vi "Save.vi"(8 "error in":errorcluster, 10 "file path":path, 11 "cRIO repo in":refnum<class "database file.lvclass">) -> (0 "error out":errorcluster, 3 "cRIO repo out":refnum<class "database file.lvclass">)   [LabVIEW 2013, in "database file.lvclass"]
doc: "Calls the Read Tree VI to have an updated version of the Repo and then saves the repo information into the XML file."
uses:
  database file.lvclass
  database file.lvclass/database file.ctl
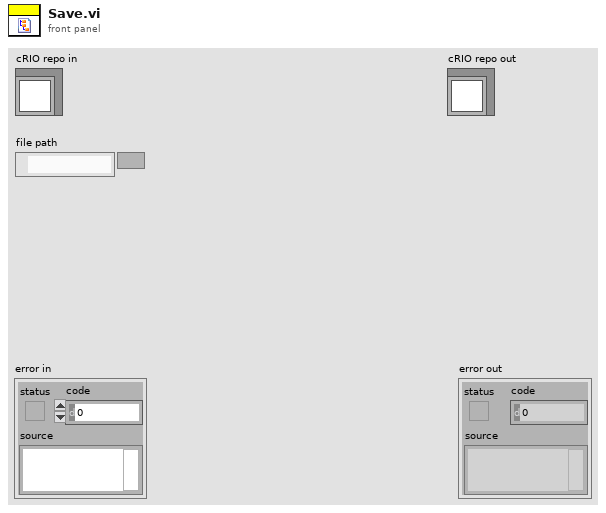
[diagram p1: front panel]
types:
  T1 = enum16{"open", "replace", "create", "open or create", "replace or create", "replace or create with confirmation"}
  T2 = typedef "J1939.lvlib/J1939 db.ctl" = cluster{"BaudRate":u32, "CAN.IoMode":u32, "J1939 Network Address":u8, "Name":u64, "frames":T3[]}
  T3 = typedef "J1939.lvlib/J1939 db frame.ctl" = cluster{"name":string, "Priority":u8, "PGN":u32, "Reserved Bit":u8, "Data page":u8, "PDU Format":u8, "PDU Specific":u8, "Source Address":u8, "PayldLen":u32, "signals":T4[], "Comment":string, "can timing type":u32, "transmit time":dbl, "direction":u16}
  T4 = typedef "J1939.lvlib/J1939 db signal.ctl" = cluster{"NameShort":string, "SPN":i32, "StartBit":u32, "NumBits":u32, "DataType":u32, "ByteOrdr":u32, "ScaleFac":dbl, "ScaleOff":dbl, "Max":dbl, "Min":dbl, "Default":dbl, "Unit":string, "Comment":string}
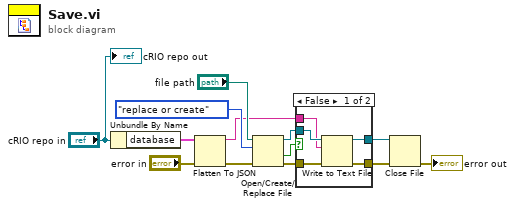
[diagram p0: block diagram]
diagram:
  n1 = Unbundle By Name("cRIO repo in") -> ("database"=w4:T2)
  n2 = Flatten To JSON(anything=w4, error in (no error)="error in") -> (JSON string=w1:string, 11:w2:errorcluster)  [unwired: 1 in]
  n3 = Open/Create/Replace File(file path (use dialog)="file path", error in=w2, operation (0:open)=T1."replace or create") -> (refnum out=w5:refnum<file>, cancelled=w8:bool, error out=w9:errorcluster)  [unwired: 3 in]
  n4 = case shown="False" w8 {
    tunnel: w9 -> [w18 w19]
    tunnel: [w17 w19] -> w7
    tunnel: [w16 w20] -> w6
    tunnel: w5 -> [w15 w20]
    tunnel: w1 -> [w14 _]
    frame False {
      n5 = Write to Text File(file (use dialog)=w15, text=w14, error in=w18) -> (refnum out=w16:refnum<file>, error out=w17:errorcluster)  [unwired: 1 in, 1 out]
    }
    frame True {
    }
  }
  n6 = Close File(refnum=w6, error in=w7) -> (error out=→"error out":errorcluster)  [unwired: 1 out]
  "cRIO repo out" <- "cRIO repo in"
